vi "Create VI Refs.vi"(8 "error in":errorcluster, 9 "Name":string, 10 "Name Library File Path":path) -> (0 "error out":errorcluster, 2 "VI Refs":T1)   [LabVIEW 2025, in "_Msg Rescript.lvlib" / "_Msg Rescript.lvclass"]
uses:
  _Msg Rescript.lvclass
  VI Refs.ctl
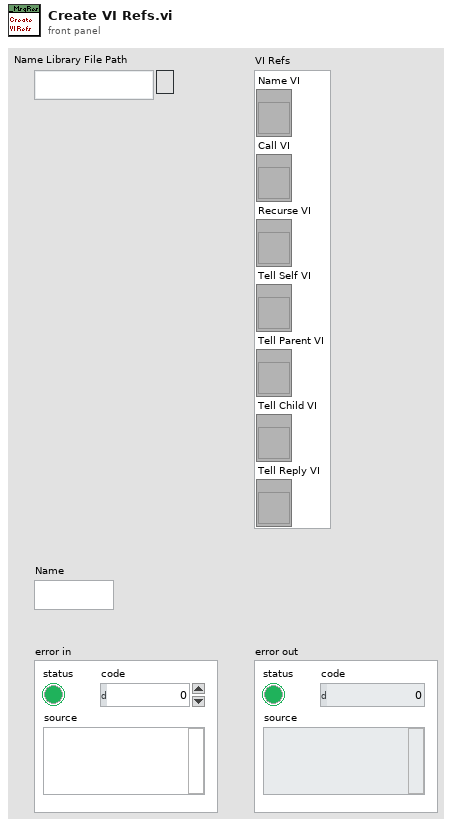
[diagram p1: front panel]
types:
  T1 = typedef "_Msg Rescript.lvlib/_Msg Rescript.lvclass/VI Refs.ctl" = cluster{"Name VI":refnum<vi>, "Call VI":refnum<vi>, "Recurse VI":refnum<vi>, "Tell Self VI":refnum<vi>, "Tell Parent VI":refnum<vi>, "Tell Child VI":refnum<vi>, "Tell Reply VI":refnum<vi>}
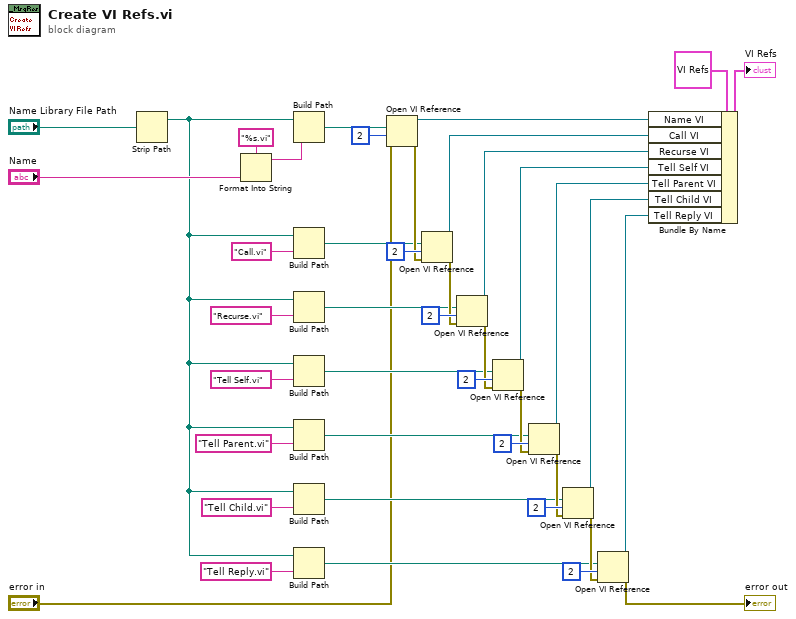
[diagram p0: block diagram]
diagram:
  n1 = Strip Path(path="Name Library File Path") -> (stripped path=w12:path)  [unwired: 1 out]
  n2 = Format Into String(format string="%s.vi", "Name") -> (resulting string=w41:string)  [unwired: 2 in, 1 out]
  n3 = Build Path(base path=w12, name or relative path=w41) -> (appended path=w40:path)
  n4 = Build Path(base path=w12, name or relative path="Call.vi" ("format string")) -> (appended path=w21:path)
  n5 = Build Path(base path=w12, name or relative path="Recurse.vi" ("format string")) -> (appended path=w20:path)
  n6 = Build Path(base path=w12, name or relative path="Tell Self.vi" ("format string")) -> (appended path=w19:path)
  n7 = Build Path(base path=w12, name or relative path="Tell Parent.vi" ("format string")) -> (appended path=w18:path)
  n8 = Build Path(base path=w12, name or relative path="Tell Child.vi" ("format string")) -> (appended path=w17:path)
  n9 = Build Path(base path=w12, name or relative path="Tell Reply.vi" ("format string")) -> (appended path=w11:path)
  n10 = Open VI Reference(vi path=w40, options=2, error in (no error)="error in") -> (vi reference=w8:refnum<vi>, error out=w31:errorcluster)  [unwired: 3 in]
  n11 = Open VI Reference(vi path=w21, options=2, error in (no error)=w31) -> (vi reference=w7:refnum<vi>, error out=w30:errorcluster)  [unwired: 3 in]
  n12 = Open VI Reference(vi path=w20, options=2, error in (no error)=w30) -> (vi reference=w6:refnum<vi>, error out=w29:errorcluster)  [unwired: 3 in]
  n13 = Open VI Reference(vi path=w19, options=2, error in (no error)=w29) -> (vi reference=w5:refnum<vi>, error out=w28:errorcluster)  [unwired: 3 in]
  n14 = Open VI Reference(vi path=w18, options=2, error in (no error)=w28) -> (vi reference=w4:refnum<vi>, error out=w27:errorcluster)  [unwired: 3 in]
  n15 = Open VI Reference(vi path=w17, options=2, error in (no error)=w27) -> (vi reference=w3:refnum<vi>, error out=w14:errorcluster)  [unwired: 3 in]
  n16 = Open VI Reference(vi path=w11, options=2, error in (no error)=w14) -> (vi reference=w2:refnum<vi>, error out=→"error out":errorcluster)  [unwired: 3 in]
  n17 = Bundle By Name(cluster=T1 {"Name VI"=refnum, "Call VI"=refnum, "Recurse VI"=refnum, "Tell Self VI"=refnum, "Tell Parent VI"=refnum, "Tell Child VI"=refnum, "Tell Reply VI"=refnum} ("VI Refs"), "Name VI"=w8, "Call VI"=w7, "Recurse VI"=w6, "Tell Self VI"=w5, "Tell Parent VI"=w4, "Tell Child VI"=w3, "Tell Reply VI"=w2) -> (→"VI Refs":T1)
